vi "Analyze Parameter File.vi"(8 "error in (no error)":errorcluster, 11 "Loop Data":T1) -> (0 "error out":errorcluster)   [LabVIEW 2016, in "System Mapping Tool.lvlib"]
uses:
  System Mapping Tool.lvlib
  TypeDefs/Model Analysis Data.ctl
  TypeDefs/Model Analysis UI Refs.ctl
  NationalInstruments.VeriStand.SystemStorageUI
  NationalInstruments.VeriStand.SystemDefinitionAPI
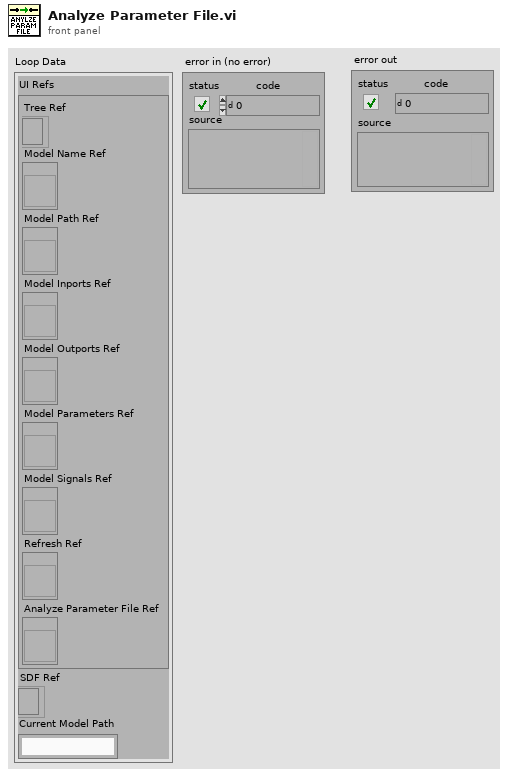
[diagram p1: front panel]
types:
  T1 = typedef "System Mapping Tool.lvlib/Model Analysis Data.ctl" = cluster{"UI Refs":T2, "SDF Ref":refnum<k24>, "Current Model Path":string}
  T2 = typedef "System Mapping Tool.lvlib/Model Analysis UI Refs.ctl" = cluster{"Tree Ref":refnum<k24>, "Model Name Ref":refnum<vi>, "Model Path Ref":refnum<vi>, "Model Inports Ref":refnum<vi>, "Model Outports Ref":refnum<vi>, "Model Parameters Ref":refnum<vi>, "Model Signals Ref":refnum<vi>, "Refresh Ref":refnum<vi>, "Analyze Parameter File Ref":refnum<vi>}
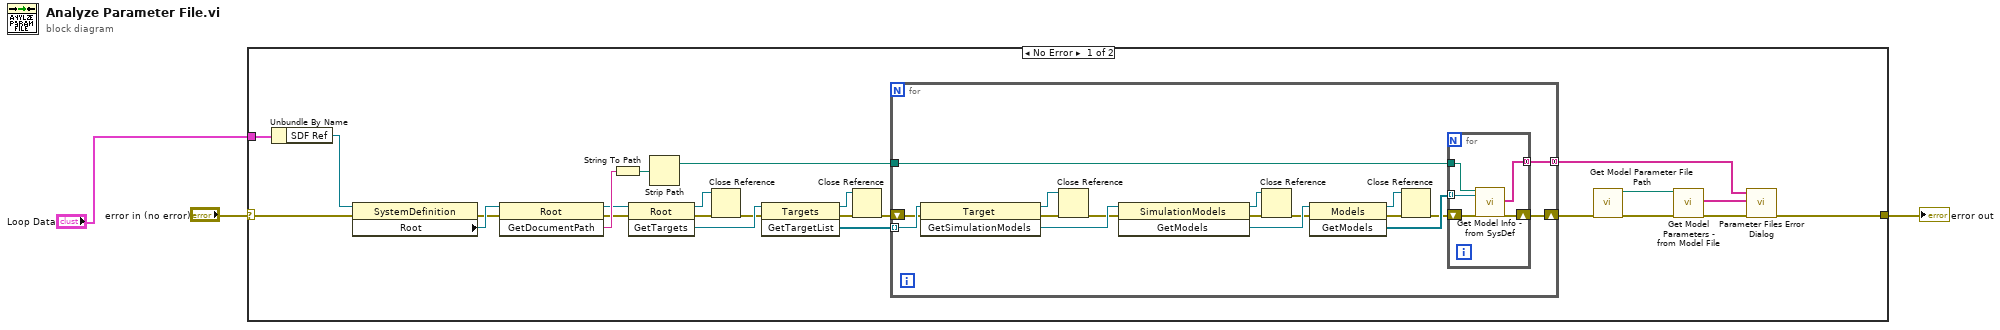
[diagram p0: block diagram]
diagram:
  n1 = case shown="No Error" "error in (no error)" {
    selector: "error in (no error)" -> [w26 w51]
    tunnel: [w20 w51] -> w2
    tunnel: "Loop Data" -> [w28 _]
    frame No Error {
      n2 = Unbundle By Name(w28) -> ("SDF Ref"=w27:refnum<k24>)
      n3 = property class="SystemDefinition"(reference=w27, error in=w26) -> (error out=w24:errorcluster, "Root"=w25:refnum<k24>)  [unwired: 1 out]
      n4 = invoke class="Root" method="GetDocumentPath"(reference=w25, error in=w24) -> (reference out=w15:refnum<k24>, error out=w16:errorcluster, "GetDocumentPath"=w23:string)  [unwired: 1 in]
      n5 = String To Path(string=w23) -> (path=w22:path)
      n6 = invoke class="Root" method="GetTargets"(reference=w15, error in=w16) -> (reference out=w11:refnum<k24>, error out=w13:errorcluster, "GetTargets"=w14:refnum<k24>)  [unwired: 1 in]
      n7 = Strip Path(path=w22) -> (stripped path=w5:path)  [unwired: 1 out]
      n8 = Close Reference(reference=w11, error in (no error)=w13) -> (error out=w12:errorcluster)
      n9 = invoke class="Targets" method="GetTargetList"(reference=w14, error in=w12) -> (reference out=w7:refnum<k24>, error out=w10:errorcluster, "GetTargetList"=w9:refnum<k24>[])  [unwired: 1 in]
      n10 = Close Reference(reference=w7, error in (no error)=w10) -> (error out=w8:errorcluster)
      n11 = for {
        shift-right: [w38] -> w6
        shift-left: w8 -> [w44]
        tunnel: w9 -> [w45] mode=indexing
        tunnel: [w33] -> w4 mode=concatenating
        tunnel: w5 -> [w31]
        n12 = invoke class="Target" method="GetSimulationModels"(reference=w45, error in=w44) -> (reference out=w41:refnum<k24>, error out=w42:errorcluster, "GetSimulationModels"=w43:refnum<k24>)  [unwired: 1 in]
        n13 = Close Reference(reference=w41, error in (no error)=w42) -> (error out=w40:errorcluster)
        n14 = invoke class="SimulationModels" method="GetModels"(reference=w43, error in=w40) -> (reference out=w30:refnum<k24>, error out=w39:errorcluster, "GetModels"=w36:refnum<k24>)  [unwired: 1 in]
        n15 = Close Reference(reference=w30, error in (no error)=w39) -> (error out=w35:errorcluster)
        n16 = invoke class="Models" method="GetModels"(reference=w36, error in=w35) -> (reference out=w29:refnum<k24>, error out=w37:errorcluster, "GetModels"=w34:refnum<k24>[])  [unwired: 1 in]
        n17 = Close Reference(reference=w29, error in (no error)=w37) -> (error out=w32:errorcluster)
        n18 = for {
          shift-right: [w49] -> w38
          shift-left: w32 -> [w50]
          tunnel: w34 -> [w48] mode=indexing
          tunnel: [w47] -> w33 mode=concatenating
          tunnel: w31 -> [w46]
          n19 = call "Get Model Info - from SysDef.vi"("System Definition Filepath (.nivssdf)"=w46, "Model Ref"=w48, "Error (in)"=w50) -> ("SysDef Parameters"=w47:string[], "Error (out)"=w49:errorcluster)  [unwired: 10 in, 5 out]
        }
      }
      n20 = call "Get Model Parameter File Path.vi"("error in (no error)"=w6) -> ("error out"=w18:errorcluster, "Model Parameter Path"=w17:path)  [unwired: 9 in]
      n21 = call "Get Model Parameters - from Model File.vi"("Model Parameter Filepath (.txt)"=w17, "Error (in)"=w18) -> ("Parameters"=w19:string[], "Error (out)"=w21:errorcluster)  [unwired: 12 in]
      n22 = call "Parameter Files Error Dialog.vi"("error in (no error)"=w21, "File Parameters"=w19, "SDF Parameters"=w4) -> ("error out"=w20:errorcluster)  [unwired: 8 in]
    }
    frame Error {
    }
  }
  "error out" <- w2
